vi "单个流程写入.vi"(7 "添加的路径":path, 8 "error in (no error)":errorcluster caption="错误输入（无错误）", 9 "量程":enum16{"低量程", "高量程"}(ring), 10 "测量模式":u16(ring) items=["", "水样测量", "标样核查", "零点核查", "跨度核查", "空白测试", "平行样测试", "加标回收", "校零", "校标"], 11 "测量参数":u16(ring)=21 items=["总磷"=0, "总氮"=1, "CODMn"=21]) -> (0 "error out":errorcluster caption="错误输出", 3 "步数":i32)   [LabVIEW 2016, in "斯坦道CODMn新电路板.lvlib"]
panel:
  out "数组 2":u16[][](array[numeric]) format="0x%04x"
  out "大小":i32
  out "交织的数组":u16[](array[numeric]) format="0x%04x"
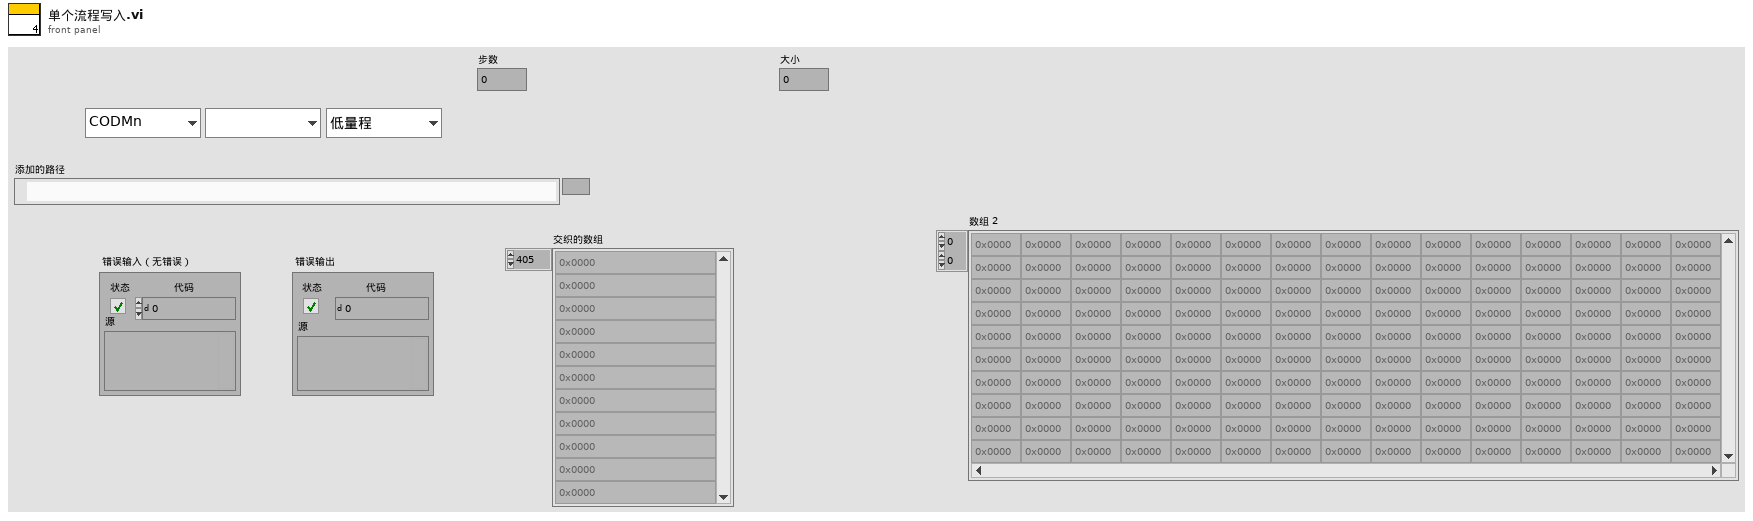
[diagram p1: front panel]
types:
  T1 = cluster{"port":u32, "pump":u16, "temp":u8, "adc":u8, "time":u16, "步骤名":string}[]
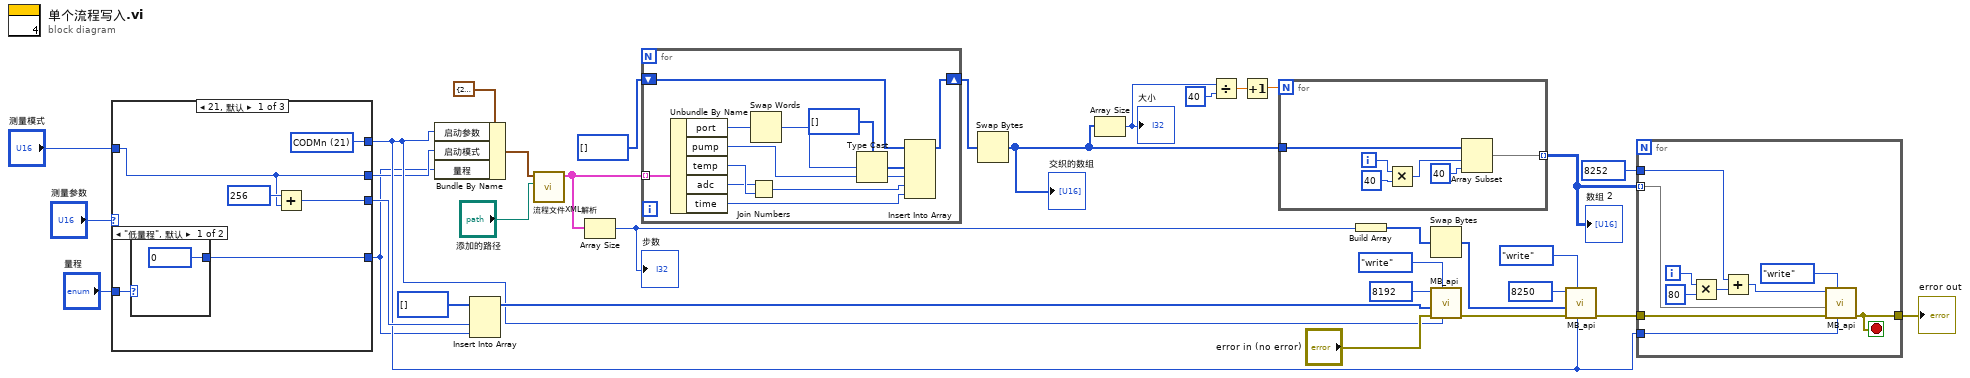
[diagram p0: block diagram]
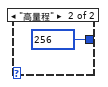
[diagram p2: hidden frame]
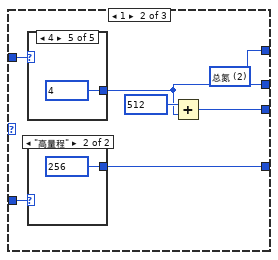
[diagram p3: hidden frame]
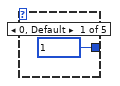
[diagram p4: hidden frame]
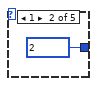
[diagram p5: hidden frame]
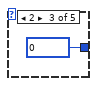
[diagram p6: hidden frame]
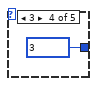
[diagram p7: hidden frame]
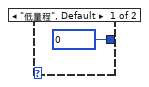
[diagram p8: hidden frame]
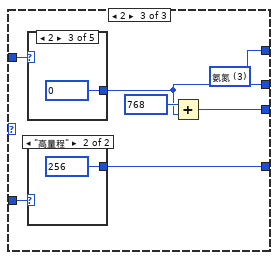
[diagram p9: hidden frame]
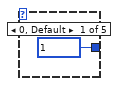
[diagram p10: hidden frame]
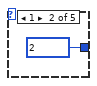
[diagram p11: hidden frame]
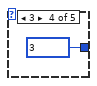
[diagram p12: hidden frame]
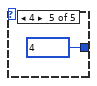
[diagram p13: hidden frame]
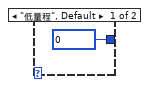
[diagram p14: hidden frame]
diagram:
  n1 = case shown="21, 默认" "测量参数" {
    tunnel: "测量模式" -> [w34 w46 w60]
    tunnel: "量程" -> [w39 w47 w61]
    tunnel: [w35 w48 w62] -> w3
    tunnel: [w36 w43 w57] -> w29
    tunnel: [w38 w45 w59] -> w1
    tunnel: [w34 w42 w56] -> w2
    frame 21, Default {
      w35 = u16 21 items=["CODMn"=21, "总氮"=2, "氨氮"=3] ("站号")
      n2 = case shown="\"低量程\", 默认" w39 {
        tunnel: [u16 0 ("starting address") u16 256 ("starting address")] -> w38
        frame "低量程", Default {
        }
        frame "高量程" {
        }
      }
      n3 = Add(x=u16 256 ("starting address"), y=w34) -> (x+y=w36:u16)
    }
    frame 1 {
      w48 = u16 2 items=["总磷"=1, "总氮"=2, "氨氮"=3] ("站号")
      n4 = case shown="4" w46 {
        tunnel: [u16 1 ("starting address") u16 2 ("starting address") u16 0 ("starting address") u16 3 ("starting address") u16 4 ("starting address")] -> w42
        frame 0, Default {
        }
        frame 1 {
        }
        frame 2 {
        }
        frame 3 {
        }
        frame 4 {
        }
      }
      n5 = case shown="\"高量程\"" w47 {
        tunnel: [u16 0 ("starting address") u16 256 ("starting address")] -> w45
        frame "低量程", Default {
        }
        frame "高量程" {
        }
      }
      n6 = Add(x=u16 512 ("starting address"), y=w42) -> (x+y=w43:u16)
    }
    frame 2 {
      w62 = u16 3 items=["总磷"=1, "总氮"=2, "氨氮"=3] ("站号")
      n7 = case shown="2" w60 {
        tunnel: [u16 1 ("starting address") u16 2 ("starting address") u16 0 ("starting address") u16 3 ("starting address") u16 4 ("starting address")] -> w56
        frame 0, Default {
        }
        frame 1 {
        }
        frame 2 {
        }
        frame 3 {
        }
        frame 4 {
        }
      }
      n8 = case shown="\"高量程\"" w61 {
        tunnel: [u16 0 ("starting address") u16 256 ("starting address")] -> w59
        frame "低量程", Default {
        }
        frame "高量程" {
        }
      }
      n9 = Add(x=u16 768 ("starting address"), y=w56) -> (x+y=w57:u16)
    }
  }
  n10 = Bundle By Name(cluster=cluster{"启动参数":u16, "启动模式":u16, "量程":u16} {"启动参数"=21, "启动模式"=1, "量程"=0} ("参数簇"), "启动参数"=w3, "启动模式"=w2, "量程"=w1) -> (w4:cluster{"启动参数":u16, "启动模式":u16, "量程":u16})
  n11 = Insert Into Array(array=u16[] [] ("数组"), new element #1=w29, new element #2=w1) -> (w23:u16[])  [unwired: 1 in]
  n12 = call "流程文件XML解析.vi"("添加的路径"="添加的路径", "参数簇"=w4) -> ("数组"=w12:T1)  [unwired: 9 in]
  n13 = Array Size(array=w12) -> (size(s)=w7:i32)
  "步数" <- w7
  n14 = for {
    tunnel: w12 -> [w81] mode=indexing
    shift-right: [w79] -> w17
    shift-left: u16[] [] -> [w77]
    n15 = Unbundle By Name(w81) -> ("port"=w74:u32, "pump"=w72:u16, "temp"=w76:u8, "adc"=w75:u8, "time"=w70:u16)
    n16 = Join Numbers(hi=w75, lo=w76) -> ((hi.lo)=w71:u16)
    n17 = Swap Words(1:w74) -> (0:w73:u32)
    n18 = Type Cast(type=u16[] [], x=w73) -> (*(type *) &x=w78:u16[])
    n19 = Insert Into Array(array=w77, new element #1=w78, new element #2=w72, new element #3=w71, new element #4=w70) -> (w79:u16[])  [unwired: 1 in]
  }
  n20 = Swap Bytes(anything=w17) -> (byte swapped=w14:u16[])
  "交织的数组" <- w14
  n21 = Array Size(array=w14) -> (size(s)=w16:i32)
  "大小" <- w16
  n22 = Divide(x=w16, y=40) -> (x/y=w10:dbl)
  n23 = Increment(x=w10) -> (x+1=w9:dbl)
  n24 = for {
    N: w9 -> [_]
    tunnel: w14 -> [w85]
    tunnel: [w82] -> w13 mode=indexing
    i -> [w87]
    n25 = Multiply(x=w87, y=40) -> (x*y=w84:i32)
    n26 = Array Subset(array=w85, index=w84, length=40 ("y")) -> (w82:u16[])
  }
  "数组 2" <- w13
  n27 = Build Array(w7) -> (w11:i32[])
  n28 = Swap Bytes(anything=w11) -> (byte swapped=w8:i32[])
  n29 = call "MB_api.vi"("Slave ID"=w3, "STEP"=enum16{"open", "read", "write", "close"}."write", "Error in"="error in (no error)", "values"=w23, "starting address"=u16 8192) -> ("error out"=w26:errorcluster)  [unwired: 4 in, 2 out]
  n30 = call "MB_api.vi"("Slave ID"=w3, "STEP"=enum16{"open", "read", "write", "close"}."write", "Error in"=w26, "values"=w8, "starting address"=u16 8250) -> ("error out"=w22:errorcluster)  [unwired: 4 in, 2 out]
  n31 = for {
    tunnel: u16 8252 ("starting address") -> [w91]
    tunnel: w22 -> [w97]
    tunnel: [w95] -> w20
    tunnel: w3 -> [w94]
    tunnel: w13 -> [w93] mode=indexing
    i -> [w90]
    stop <- w95 stop-if-true
    n32 = Multiply(x=w90, y=80) -> (x*y=w89:i32)
    n33 = Add(x=w91, y=w89) -> (x+y=w92:i32)
    n34 = call "MB_api.vi"("Slave ID"=w94, "STEP"=enum16{"open", "read", "write", "close"}."write", "Error in"=w97, "values"=w93, "starting address"=w92) -> ("error out"=w95:errorcluster)  [unwired: 4 in, 2 out]
  }
  "error out" <- w20
